vi "AngleFinder.vi"(2 "Initial Speed(in/s)":dbl, 3 "Vision Distance(in)":dbl) -> (0 "error out":errorcluster, 1 "Angle(degrees)":dbl)   [LabVIEW 2015]
doc: "Returns the angle required to score a high goal for a given launch speed, or an error if the speed is not fast enough to score."
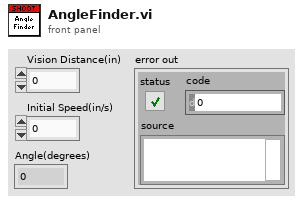
[diagram p1: front panel]
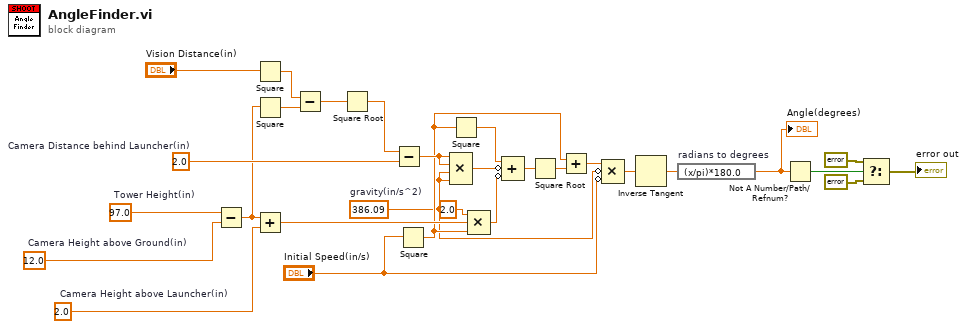
[diagram p0: block diagram]
diagram:
  w17 = 2.0  # Camera Height above Launcher(in)
  w5 = 386.09  # gravity(in/s^2)
  w29 = 2.0  # Camera Distance behind Launcher(in)
  w27 = 12.0  # Camera Height above Ground(in)
  w28 = 97.0  # Tower Height(in)
  n1 = Subtract(x=w28, y=w27) -> (x-y=w16:dbl)
  n2 = Square(x="Vision Distance(in)") -> (x^2=w23:dbl)
  n3 = Square(x=w16) -> (x^2=w24:dbl)
  n4 = Add(x=w16, y=w17) -> (x+y=w11:dbl)
  n5 = Subtract(x=w23, y=w24) -> (x-y=w25:dbl)
  n6 = Square Root(x=w25) -> (sqrt(x)=w22:dbl)
  n7 = Subtract(x=w22, y=w29) -> (x-y=w13:dbl)
  n8 = Square(x="Initial Speed(in/s)") -> (x^2=w9:dbl)
  n9 = Compound Arithmetic op=MULTIPLY(w13, w13, w5, w5) -> (w14:dbl)
  n10 = Square(x=w9) -> (x^2=w15:dbl)
  n11 = Compound Arithmetic op=MULTIPLY(2.0 ("value"), w11, w9) -> (w10:dbl)
  n12 = Compound Arithmetic op=ADD(w15, invert w14, invert w10) -> (w8:dbl)
  n13 = Square Root(x=w8) -> (sqrt(x)=w7:dbl)
  n14 = Add(x=w9, y=w7) -> (x+y=w6:dbl)
  n15 = Compound Arithmetic op=MULTIPLY(w6, invert w5, invert "Initial Speed(in/s)") -> (w3:dbl)
  n16 = Inverse Tangent(1:w3) -> (0:w2:dbl)
  n17 = expression code="(x/pi)*180.0" "radians to degrees"(w2) -> (w1:dbl)
  "Angle(degrees)" <- w1
  n18 = Not A Number/Path/Refnum?(number/path/refnum=w1) -> (NaN/Path/Refnum?=w21:bool)
  n19 = Select(t=errorcluster {"status"=TRUE, "code"=9001, "source"="Speed not fast enough to score ball at this distance!"} ("error constant"), s=w21, f=errorcluster {"status"=FALSE, "code"=0, "source"=""}) -> (s? t:f=→"error out":errorcluster)
